vi "Get 2D Picture Ring from Map.vi"(8 "error in (no error)":errorcluster, 11 "Grassfire in":refnum<class "Grassfire.lvclass">) -> (0 "error out":errorcluster, 2 "Array":T1[][](array[typedef]), 3 "Grassfire out":refnum<class "Grassfire.lvclass">)   [LabVIEW 2019, in "Grassfire.lvclass"]
uses:
  Grassfire.lvclass
  Solution--cluster.ctl
  Solution--picture ring.ctl
  Grassfire.lvclass/Grassfire.ctl
  Address/Address.lvclass/Address.ctl
  Node/Node Value.lvclass/Node Value.ctl
  Node/Read Distance.vi
  Node/Read Node Type.vi
  Address/Read Row.vi
  Address/Read Column.vi
  Address/Address.lvclass
  Node/Node Value.lvclass
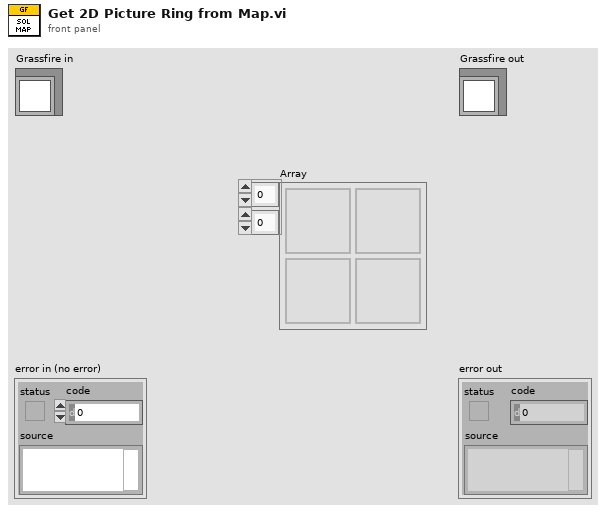
[diagram p1: front panel]
types:
  T1 = typedef "Grassfire.lvclass/Solution--cluster.ctl" = cluster{"Node Type":T2, "Distance":string}
  T2 = typedef "Grassfire.lvclass/Solution--picture ring.ctl" = i64
  T3 = map{refnum<class "Address.lvclass">, refnum<class "Node Value.lvclass">}
  T4 = typedef "Picture Ring.lvclass/Node Type--enum.ctl" = enum16{"Empty", "Blocked", "Start", "End", "Path"}
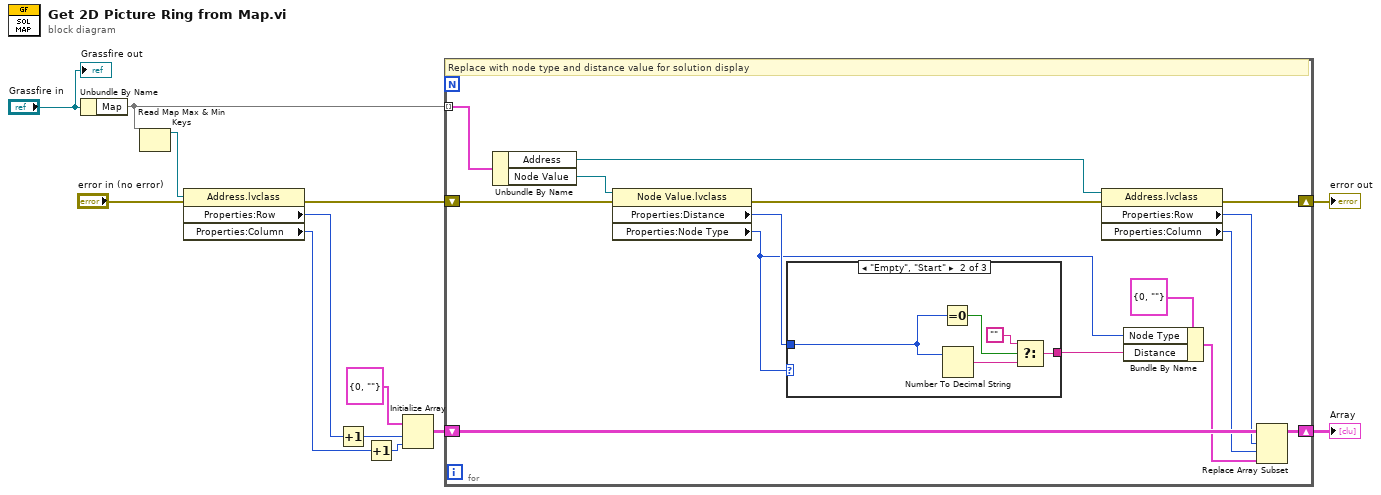
[diagram p0: block diagram]
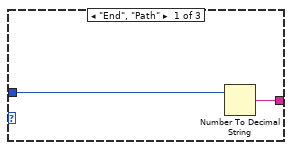
[diagram p2: hidden frame]
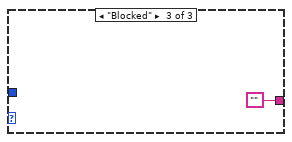
[diagram p3: hidden frame]
diagram:
  n1 = Unbundle By Name("Grassfire in") -> ("Map"=w6:T3)
  n2 = Read Map Max & Min Keys(11:w6) -> (3:w13:refnum<class "Address.lvclass">)  [unwired: 1 out]
  n3 = property class="Address.lvclass"(reference=w13, error in="error in (no error)") -> (error out=w3:errorcluster, "Properties:Row"=w12:i32, "Properties:Column"=w11:i32)  [unwired: 1 out]
  n4 = Increment(x=w12) -> (x+1=w10:i32)
  n5 = Increment(x=w11) -> (x+1=w9:i32)
  n6 = Initialize Array(T1 {"Node Type"=0, "Distance"=""} ("Node"), w10, w9) -> (w7:T1[][])
  n7 = for {
    shift-right: [w26] -> w1
    shift-left: w7 -> [w27]
    tunnel: w6 -> [w28] mode=indexing
    shift-right: [w19] -> w2
    shift-left: w3 -> [w21]
    # "Replace with node type and distance value for solution display"
    n8 = Unbundle By Name(w28) -> ("Address"=w25:refnum<class "Address.lvclass">, "Node Value"=w22:refnum<class "Node Value.lvclass">)
    n9 = property class="Node Value.lvclass"(reference=w22, error in=w21) -> (error out=w20:errorcluster, "Properties:Distance"=w18:i32, "Properties:Node Type"=w14:T4)  [unwired: 1 out]
    n10 = case shown="\"Empty\", \"Start\"" w14 {
      tunnel: w18 -> [w30 w35 _]
      tunnel: [w29 w31 ""] -> w15
      frame "End", "Path" {
        n11 = Number To Decimal String(number=w30) -> (decimal integer string=w29:string)  [unwired: 1 in]
      }
      frame "Empty", "Start" {
        n12 = Equal To 0?(x=w35) -> (x = 0?=w34:bool)
        n13 = Number To Decimal String(number=w35) -> (decimal integer string=w32:string)  [unwired: 1 in]
        n14 = Select(t="", s=w34, f=w32) -> (s? t:f=w31:string)
      }
      frame "Blocked" {
      }
    }
    n15 = property class="Address.lvclass"(reference=w25, error in=w20) -> (error out=w19:errorcluster, "Properties:Row"=w24:i32, "Properties:Column"=w23:i32)  [unwired: 1 out]
    n16 = Bundle By Name(cluster=T1 {"Node Type"=0, "Distance"=""} ("Node"), "Node Type"=w14, "Distance"=w15) -> (w16:T1)
    n17 = Replace Array Subset(array=w27, new element=w16, index (row)=w24, index (col)=w23) -> (w26:T1[][])
  }
  "error out" <- w2
  "Array" <- w1
  "Grassfire out" <- "Grassfire in"
